vi "get_attribute_from_string_ID.vi"(8 "error in":errorcluster caption="error in (no error)", 10 "Attribute ID in":string, 11 "VISA resource name":refnum<visa-resource-name>) -> (0 "error out":errorcluster, 2 "Attribute out":T1={"Identifier"="", "Descriptive Name"="", "Data Type"=enum."Integer 32", "Command"="", "Access"=enum."Read/Write", "Range Table"="", "Read Callback"="", "Write Callback"="", "Supported Models"="", "Instrument Options"="", "Index"=0, "OPC Wait"=FALSE, "No Status Check"=FALSE, "Cache Only"=FALSE}, 3 "VISA resource name out":refnum<visa-resource-name>)   [LabVIEW 2020, in "Rohde&Schwarz RTx Oscilloscopes.lvlib" / "rsidr_core.lvlib"]
uses:
  rsidr_core.lvlib
  type_Attribute.ctl
  type_Attribute_Data_Type.ctl
  type_ReadWriteAccess.ctl
  _type_Operation_Fgv_Attributes.ctl
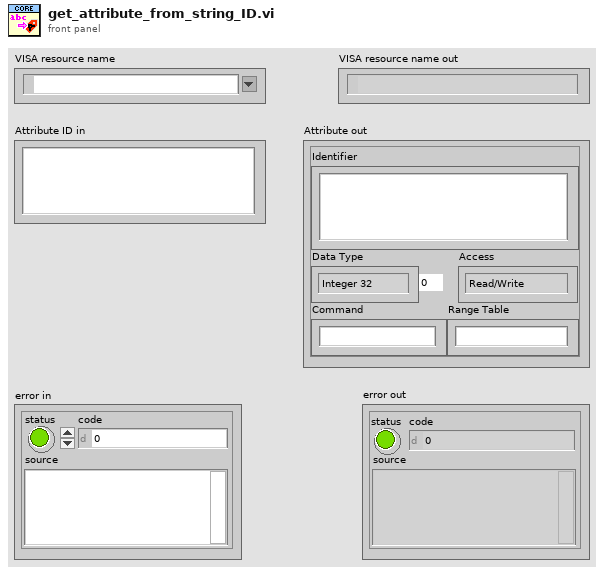
[diagram p1: front panel]
types:
  T1 = typedef "Rohde&Schwarz RTx Oscilloscopes.lvlib/rsidr_core.lvlib/type_Attribute.ctl" = cluster{"Identifier":string, "Descriptive Name":string, "Data Type":T2, "Command":string, "Access":T3, "Range Table":string, "Read Callback":string, "Write Callback":string, "Supported Models":string, "Instrument Options":string, "Index":i32, "OPC Wait":bool, "No Status Check":bool, "Cache Only":bool}
  T2 = typedef "Rohde&Schwarz RTx Oscilloscopes.lvlib/rsidr_core.lvlib/type_Attribute_Data_Type.ctl" = enum16{"Integer 32", "Double", "String", "Boolean", "None", "Integer 64", "RawString"}
  T3 = typedef "Rohde&Schwarz RTx Oscilloscopes.lvlib/rsidr_core.lvlib/type_ReadWriteAccess.ctl" = enum16{"Read Only", "Write Only", "Read/Write"}
  T4 = typedef "Rohde&Schwarz RTx Oscilloscopes.lvlib/rsidr_core.lvlib/_type_Operation_Fgv_Attributes.ctl" = enum16{"Initialize", "Get Attribute"}
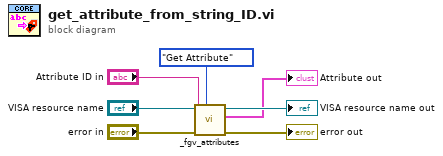
[diagram p0: block diagram]
diagram:
  n1 = call "_fgv_attributes.vi"("Operation"=_type_Operation_Fgv_Attributes."Get Attribute", "error in"="error in", "Attribute ID in"="Attribute ID in", "VISA resource name"="VISA resource name") -> ("error out"=→"error out":errorcluster, "Attribute out"=→"Attribute out":T1, "VISA resource name out"=→"VISA resource name out":refnum<visa-resource-name>)  [unwired: 4 in, 1 out]
